vi "Configure Keithley DMM7510.vi"(6 "Sampling interval [s]":dbl=1e-05, 7 "Manual Range":dbl=10.0, 8 "error in (no error)":errorcluster, 9 "Coupling":T2 items=["AC", "DC"], 10 "Quantity":T1 items=["Voltage", "Current"], 11 "VISA resource name":refnum<visa-resource-name>) -> (0 "error out":errorcluster, 3 "VISA resource name out":refnum<visa-resource-name>)   [LabVIEW 2016, in "Acquisition.lvlib"]
uses:
  Acquisition/Acquisition.lvlib
  Settings/Coupling.ctl
  Settings/Quantity.ctl
  Keithley DMM7510.lvlib
  Settings/Settings.lvlib
panel:
  in  "Auto Zero State":bool
  in  "Bandwidth (30)":u16(ring)=2 items=["3", "30", "300"]
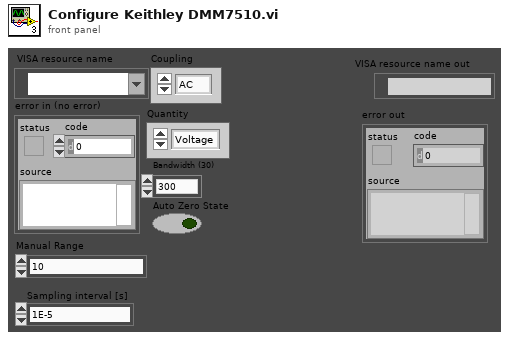
[diagram p1: front panel]
types:
  T1 = typedef "Settings.lvlib/Quantity.ctl" = u16
  T2 = typedef "Settings.lvlib/Coupling.ctl" = i16
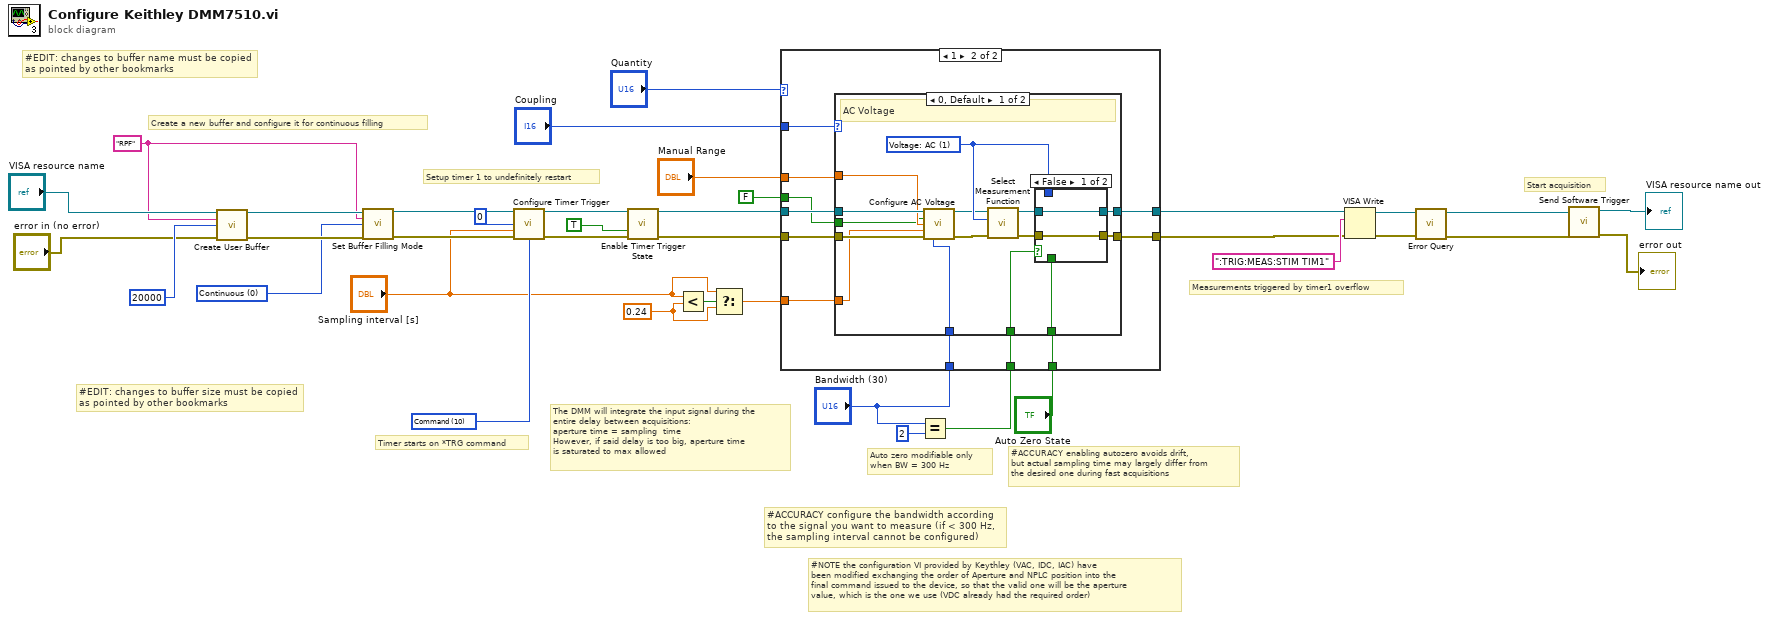
[diagram p0: block diagram]
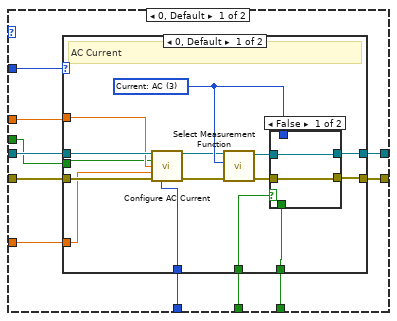
[diagram p2: hidden frame]
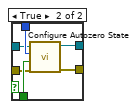
[diagram p3: hidden frame]
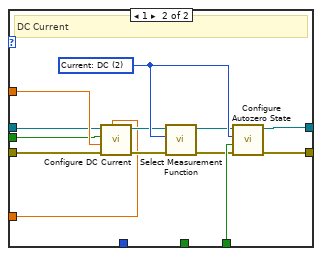
[diagram p4: hidden frame]
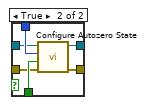
[diagram p5: hidden frame]
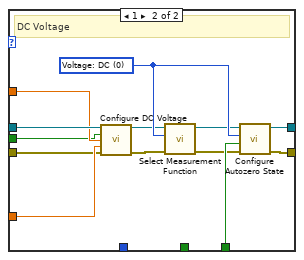
[diagram p6: hidden frame]
diagram:
  w35 = 0.24 ("y")
  w24 = u16 10 items=["None", "Front Pannel Trigger Key", "Notify Trigger Block 1", "Notify Trigger Block 2", "Notify Trigger Block 3", "Notify Trigger Block 4", "Notify Trigger Block 5", "Notify Trigger Block 6", "Notify Trigger Block 7", "Notify Trigger Block 8", "Command", "Digi IO Line 1", "Digi IO Line 2", "Digi IO Line 3", "Digi IO Line 4", "Digi IO Line 5", "Digi IO Line 6", "TSP-Link 1", "TSP-Link 2", "TSP-Link 3", "LAN 1", "LAN 2", "LAN 3", "LAN 4", "LAN 5", "LAN 6", "LAN 7", "LAN 8", "Blender 1", "Blender 2", "Timer 1", "Timer 2", "Timer 3", "Timer 4", "Analog Trigger", "External Trigger"] ("Stimulus Event")
  w28 = u16 0 items=["Continuous", "Once"] ("Fill Type")
  w29 = "RPF" ("Buffer Name")
  # "Auto zero modifiable only\nwhen BW = 300 Hz"
  # "#NOTE the configuration VI provided by Keythley (VAC, IDC, IAC) have\nbeen modified exchanging the order of Aperture and NPLC position into the\nfinal command issued to the device, so that the valid one will be the aperture\nvalue, which is the one we use (VDC already had the required order)"
  # "#EDIT: changes to buffer name must be copied\nas pointed by other bookmarks"
  # "#EDIT: changes to buffer size must be copied\nas pointed by other bookmarks"
  # "#ACCURACY configure the bandwidth according\nto the signal you want to measure (if < 300 Hz,\nthe sampling interval cannot be configured)"
  # "#ACCURACY enabling autozero avoids drift,\nbut actual sampling time may largely differ from\nthe desired one during fast acquisitions"
  # "Start acquisition"
  # "The DMM will integrate the input signal during the\nentire delay between acquisitions: \naperture time = sampling  time\nHowever, if said delay is too big, aperture time\nis saturated to max allowed"
  # "Measurements triggered by timer1 overflow"
  # "Setup timer 1 to undefinitely restart"
  # "Create a new buffer and configure it for continuous filling"
  # "Timer starts on *TRG command"
  n1 = call "Create User Buffer.vi"("VISA resource name"="VISA resource name", "Buffer Name"=w29, "Buffer Size"=20000, "error in (no error)"="error in (no error)") -> ("VISA resource name out"=w30:refnum<visa-resource-name>, "error out"=w31:errorcluster)  [unwired: 10 in]
  n2 = call "Set Buffer Filling Mode.vi"("VISA resource name"=w30, "Buffer Name (defbuffer1)"=w29, "Fill Type"=w28, "error in (no error)"=w31) -> ("VISA resource name out"=w27:refnum<visa-resource-name>, "error out"=w26:errorcluster)  [unwired: 10 in]
  n3 = call "Configure Timer Trigger.vi"("VISA resource name"=w27, "Count"=0, "Delay"="Sampling interval [s]", "error in (no error)"=w26, "Stimulus Event"=w24) -> ("VISA resource name out"=w21:refnum<visa-resource-name>, "error out"=w23:errorcluster)  [unwired: 9 in]
  n4 = call "Enable Timer Trigger State.vi"("VISA resource name"=w21, "Enable Beeper"=TRUE, "error in (no error)"=w23) -> ("VISA resource name out"=w20:refnum<visa-resource-name>, "error out"=w17:errorcluster)  [unwired: 11 in]
  n5 = Less?(x="Sampling interval [s]", y=w35) -> (x < y?=w36:bool)
  n6 = Select(t="Sampling interval [s]", s=w36, f=w35) -> (s? t:f=w18:dbl)
  n7 = Equal?(x="Bandwidth (30)", y=u16 2) -> (x = y?=w1:bool)
  n8 = case shown="1" "Quantity" {
    tunnel: w20 -> [w43 w95]
    tunnel: "Manual Range" -> [w44 w94]
    tunnel: w18 -> [w41 w93]
    tunnel: w17 -> [w42 w92]
    tunnel: [w46 w91] -> w16
    tunnel: [w47 w90] -> w15
    tunnel: "Coupling" -> [w45 w89]
    tunnel: FALSE ("Auto Range? (T: Auto)") -> [w40 w86]
    tunnel: "Bandwidth (30)" -> [w39 w88]
    tunnel: "Auto Zero State" -> [w48 w87]
    tunnel: w1 -> [w38 w85]
    frame 0, Default {
      n9 = case shown="0, Default" w45 {
        tunnel: w43 -> [w63 w79]
        tunnel: w44 -> [w61 w84]
        tunnel: w41 -> [w60 w72]
        tunnel: w42 -> [w62 w83]
        tunnel: [w57 w81] -> w46
        tunnel: [w58 w82] -> w47
        tunnel: w39 -> [w59 _]
        tunnel: w48 -> [w56 w80]
        tunnel: w40 -> [w55 w78]
        tunnel: w38 -> [w49 _]
        frame 0, Default {
          w54 = u16 3 items=["Voltage: DC", "Voltage: AC", "Current: DC", "Current: AC", "2W Resistance", "4W Resistance", "Diode", "Capacitance", "Temperature", "Continuity", "Frequency", "Period", "Ratio", "Digitize Voltage", "Digitize Current"] ("Function")
          # "AC Current"
          n10 = call "Configure AC Current.vi"("VISA resource name"=w63, "Auto Range? (T: Auto)"=w55, "Manual Range"=w61, "Aperture Seconds"=w60, "error in (no error)"=w62, "Bandwidth (30)"=w59) -> ("VISA resource name out"=w53:refnum<visa-resource-name>, "error out"=w52:errorcluster)  [unwired: 8 in]
          n11 = call "Select Measurement Function.vi"("error in (no error)"=w52, "Function"=w54, "VISA resource name"=w53) -> ("error out"=w51:errorcluster, "VISA resource name out"=w50:refnum<visa-resource-name>)  [unwired: 7 in]
          n12 = case shown="False" w49 {
            tunnel: [w65 w71] -> w58
            tunnel: [w64 w70] -> w57
            tunnel: w56 -> [_ w69]
            tunnel: w54 -> [_ w68]
            tunnel: w51 -> [w64 w67]
            tunnel: w50 -> [w65 w66]
            frame False {
            }
            frame True {
              n13 = call "Configure Autozero State.vi"("error in (no error)"=w67, "Auto Zero State"=w69, "Function"=w68, "VISA resource name"=w66) -> ("error out"=w70:errorcluster, "VISA resource name out"=w71:refnum<visa-resource-name>)  [unwired: 6 in]
            }
          }
        }
        frame 1 {
          w77 = u16 2 items=["Voltage: DC", "Voltage: AC", "Current: DC", "Current: AC", "2W Resistance", "4W Resistance", "Diode", "Capacitance", "Temperature", "Continuity", "Frequency", "Period", "Ratio", "Digitize Voltage", "Digitize Current"] ("Function")
          # "DC Current"
          n14 = call "Configure DC Current.vi"("Aperture Seconds"=w72, "error in (no error)"=w83, "Manual Range"=w84, "Auto Range? (T: Auto)"=w78, "VISA resource name"=w79) -> ("error out"=w76:errorcluster, "VISA resource name out"=w75:refnum<visa-resource-name>)  [unwired: 5 in]
          n15 = call "Select Measurement Function.vi"("error in (no error)"=w76, "Function"=w77, "VISA resource name"=w75) -> ("error out"=w73:errorcluster, "VISA resource name out"=w74:refnum<visa-resource-name>)  [unwired: 7 in]
          n16 = call "Configure Autozero State.vi"("error in (no error)"=w73, "Auto Zero State"=w80, "Function"=w77, "VISA resource name"=w74) -> ("error out"=w81:errorcluster, "VISA resource name out"=w82:refnum<visa-resource-name>)  [unwired: 6 in]
        }
      }
    }
    frame 1 {
      n17 = case shown="0, Default" w89 {
        tunnel: w95 -> [w110 w131]
        tunnel: w94 -> [w108 w130]
        tunnel: w93 -> [w98 w129]
        tunnel: w92 -> [w109 w128]
        tunnel: [w106 w126] -> w91
        tunnel: [w107 w127] -> w90
        tunnel: w88 -> [w97 _]
        tunnel: w87 -> [w105 w125]
        tunnel: w86 -> [w104 w124]
        tunnel: w85 -> [w96 _]
        frame 0, Default {
          w103 = u16 1 items=["Voltage: DC", "Voltage: AC", "Current: DC", "Current: AC", "2W Resistance", "4W Resistance", "Diode", "Capacitance", "Temperature", "Continuity", "Frequency", "Period", "Ratio", "Digitize Voltage", "Digitize Current"] ("Function")
          # "AC Voltage"
          n18 = call "Configure AC Voltage.vi"("VISA resource name"=w110, "Auto Range? (T: Auto)"=w104, "Manual Range"=w108, "Aperture Seconds"=w98, "error in (no error)"=w109, "Bandwidth (30)"=w97) -> ("VISA resource name out"=w102:refnum<visa-resource-name>, "error out"=w101:errorcluster)  [unwired: 8 in]
          n19 = call "Select Measurement Function.vi"("error in (no error)"=w101, "Function"=w103, "VISA resource name"=w102) -> ("error out"=w99:errorcluster, "VISA resource name out"=w100:refnum<visa-resource-name>)  [unwired: 7 in]
          n20 = case shown="False" w96 {
            tunnel: [w112 w118] -> w107
            tunnel: [w111 w117] -> w106
            tunnel: w105 -> [_ w116]
            tunnel: w103 -> [_ w115]
            tunnel: w100 -> [w112 w114]
            tunnel: w99 -> [w111 w113]
            frame False {
            }
            frame True {
              n21 = call "Configure Autozero State.vi"("error in (no error)"=w113, "Auto Zero State"=w116, "Function"=w115, "VISA resource name"=w114) -> ("error out"=w117:errorcluster, "VISA resource name out"=w118:refnum<visa-resource-name>)  [unwired: 6 in]
            }
          }
        }
        frame 1 {
          w123 = u16 0 items=["Voltage: DC", "Voltage: AC", "Current: DC", "Current: AC", "2W Resistance", "4W Resistance", "Diode", "Capacitance", "Temperature", "Continuity", "Frequency", "Period", "Ratio", "Digitize Voltage", "Digitize Current"] ("Function")
          # "DC Voltage"
          n22 = call "Configure DC Voltage.vi"("VISA resource name"=w131, "Auto Range? (T: Auto)"=w124, "Manual Range"=w130, "Aperture Seconds"=w129, "error in (no error)"=w128) -> ("VISA resource name out"=w122:refnum<visa-resource-name>, "error out"=w121:errorcluster)  [unwired: 9 in]
          n23 = call "Select Measurement Function.vi"("error in (no error)"=w121, "Function"=w123, "VISA resource name"=w122) -> ("error out"=w119:errorcluster, "VISA resource name out"=w120:refnum<visa-resource-name>)  [unwired: 7 in]
          n24 = call "Configure Autozero State.vi"("error in (no error)"=w119, "Auto Zero State"=w125, "Function"=w123, "VISA resource name"=w120) -> ("error out"=w126:errorcluster, "VISA resource name out"=w127:refnum<visa-resource-name>)  [unwired: 6 in]
        }
      }
    }
  }
  n25 = VISA Write(VISA resource name=w15, write buffer=":TRIG:MEAS:STIM TIM1", error in (no error)=w16) -> (VISA resource name out=w14:refnum<visa-resource-name>, error out=w13:errorcluster)  [unwired: 1 out]
  n26 = call "Error Query.vi"("error in (no error)"=w13, "VISA resource name"=w14) -> ("error out"=w8:errorcluster, "VISA resource name out"=w9:refnum<visa-resource-name>)  [unwired: 6 in, 2 out]
  n27 = call "Send Software Trigger.vi"("error in (no error)"=w8, "VISA resource name"=w9) -> ("error out"=→"error out":errorcluster, "VISA resource name out"=→"VISA resource name out":refnum<visa-resource-name>)  [unwired: 8 in]
